vi "ParamSetAll.vi"(10 "error in (no error)":errorcluster caption="错误输入（无错误）") -> ()   [LabVIEW 2018]
panel:
  in  "确定":bool
  out "数值":i32
  out "原始数据":string[](array[string])=["general_param.vi", "PowerEnergyMeter_param.vi", "SpecMeter_param.vi", "Scope_param.vi", "Polarmeter_param.vi", "NearFieldCamera_param.vi", "FarFieldCamera_param.vi"]
  # "参数设置完成后，点击确定，参数下次运行会自动加载"
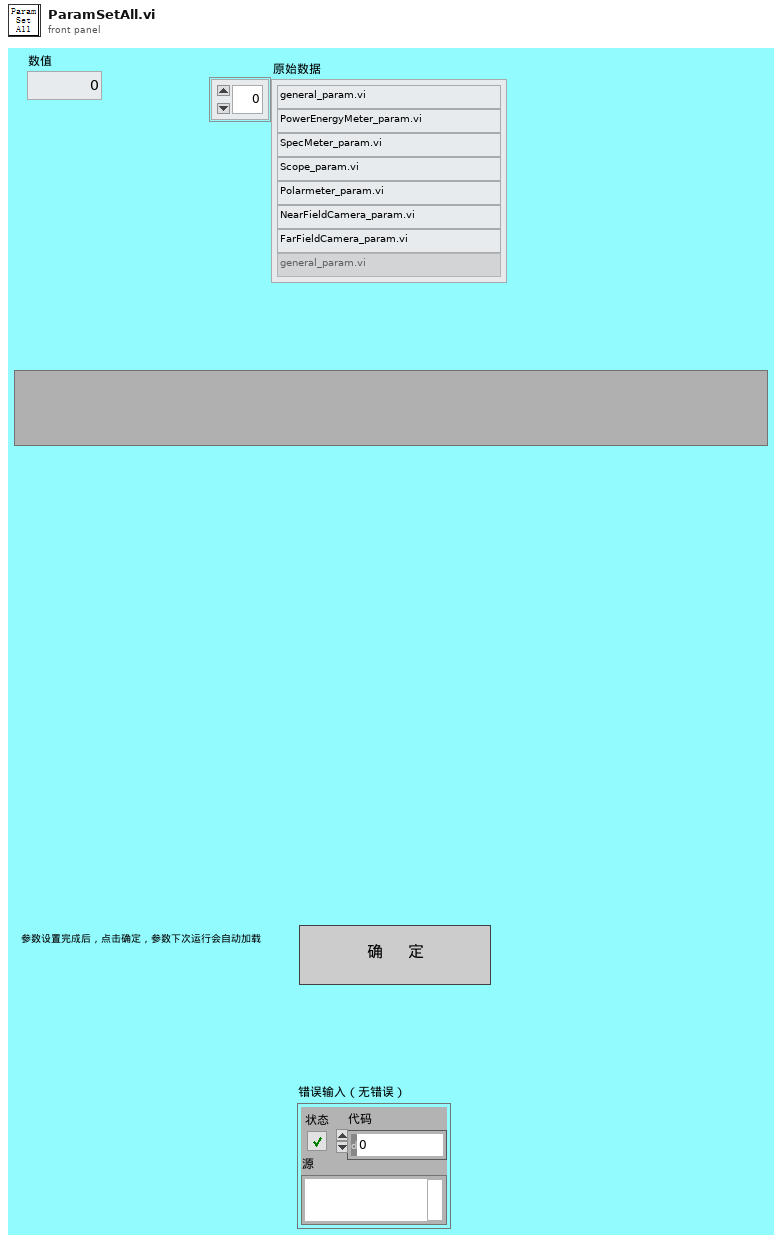
[diagram p1: front panel]
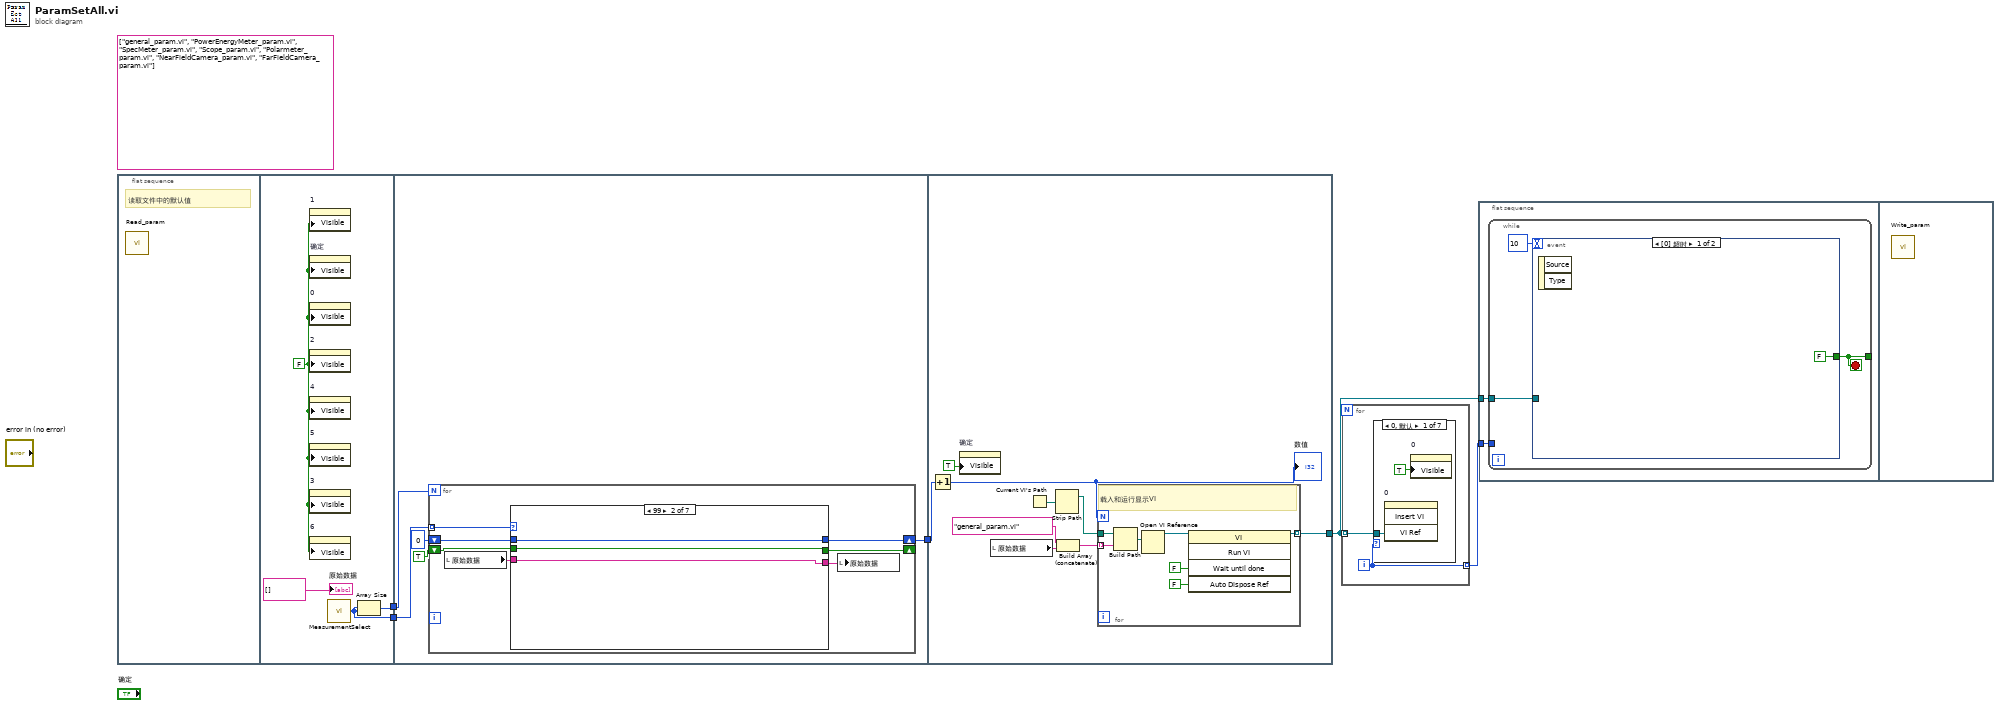
[diagram p0: block diagram]
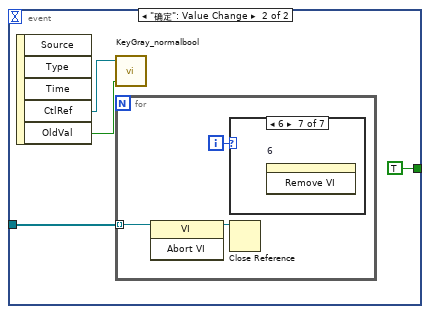
[diagram p2: hidden frame]
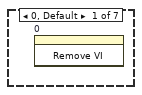
[diagram p3: hidden frame]
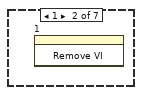
[diagram p4: hidden frame]
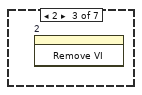
[diagram p5: hidden frame]
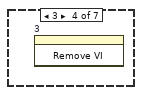
[diagram p6: hidden frame]
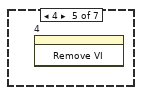
[diagram p7: hidden frame]
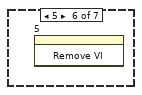
[diagram p8: hidden frame]
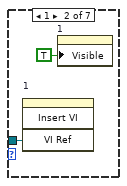
[diagram p9: hidden frame]
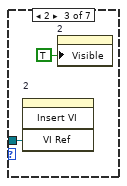
[diagram p10: hidden frame]
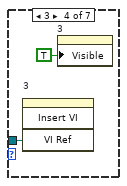
[diagram p11: hidden frame]
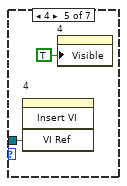
[diagram p12: hidden frame]
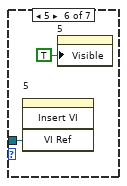
[diagram p13: hidden frame]
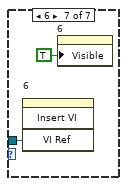
[diagram p14: hidden frame]
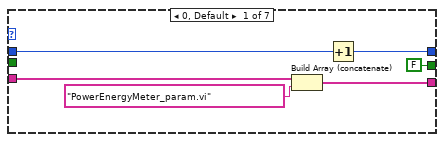
[diagram p15: hidden frame]
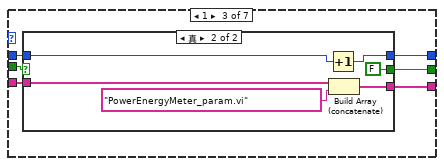
[diagram p16: hidden frame]
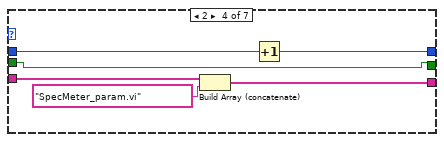
[diagram p18: hidden frame]
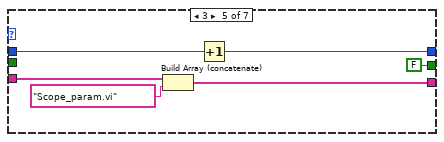
[diagram p19: hidden frame]
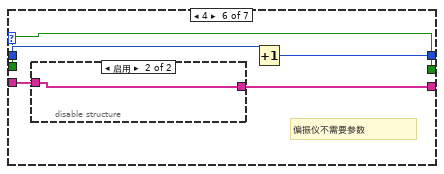
[diagram p20: hidden frame]
diagram:
  (unwired) string[] ["general_param.vi", "PowerEnergyMeter_param.vi", "SpecMeter_param.vi", "Scope_param.vi", "Polarmeter_param.vi", "NearFieldCamera_param.vi", "FarFieldCamera_param.vi"]
  n1 = flat-sequence {
    tunnel: [w8] -> w2
    tunnel: [w7] -> w1
    tunnel: [w12] -> w5
    tunnel: w2 -> [w11]
    tunnel: w1 -> [w10]
    tunnel: w5 -> [w81]
    tunnel: [w77] -> w3
    frame #0 {
      # "读取文件中的默认值"
      n2 = call "Read_param.vi"() -> ()  [unwired: 12 in]
    }
    frame #1 {
      w6 = FALSE
      n3 = property on="1" class="SubPnl"("Visible"=w6) -> ()  [unwired: 2 in, 2 out]
      n4 = property on="确定" class="Bool (严格)"("Visible"=w6) -> ()  [unwired: 2 in, 2 out]
      n5 = property on="0" class="SubPnl"("Visible"=w6) -> ()  [unwired: 2 in, 2 out]
      n6 = property on="2" class="SubPnl"("Visible"=w6) -> ()  [unwired: 2 in, 2 out]
      n7 = property on="4" class="SubPnl"("Visible"=w6) -> ()  [unwired: 2 in, 2 out]
      n8 = property on="5" class="SubPnl"("Visible"=w6) -> ()  [unwired: 2 in, 2 out]
      n9 = property on="3" class="SubPnl"("Visible"=w6) -> ()  [unwired: 2 in, 2 out]
      n10 = property on="6" class="SubPnl"("Visible"=w6) -> ()  [unwired: 2 in, 2 out]
      n11 = call "MeasurementSelect.vi"() -> ("任务序号"=w7:i32[])  [unwired: 1 in]
      n12 = Array Size(array=w7) -> (size(s)=w8:i32)
      "原始数据" <- string[] []
    }
    frame #2 {
      n13 = for {
        N: w11 -> [_]
        shift-right: [w20] -> _
        shift-left: TRUE -> [w21]
        shift-right: [w18] -> w12
        shift-left: 0 -> [w19]
        tunnel: w10 -> [w17] mode=indexing
        n14 = local read "原始数据"() -> (w15:string[])
        n15 = case shown="99" w17 {
          tunnel: w21 -> [_ w29 w36 w51 _ w60 w71]
          tunnel: [FALSE w29 w32 w51 FALSE w60 w71] -> w20
          tunnel: [w22 w30 w35 w46 w52 w58 w67] -> w16
          tunnel: w19 -> [w26 w28 w34 w50 w56 w62 w74]
          tunnel: [w25 w28 w33 w49 w55 w61 w72] -> w18
          tunnel: w15 -> [w24 w30 w31 w48 w54 w59 w70]
          frame 0, Default {
            n16 = Build Array (concatenate)(w24, "PowerEnergyMeter_param.vi" ("名称或相对路径")) -> (w22:string[])
            n17 = Increment(x=w26) -> (x+1=w25:i32)
          }
          frame 99 {
          }
          frame 1 {
            n18 = case shown="真" w36 {
              selector: w36 -> [w38 _]
              tunnel: [w37 w41] -> w35
              tunnel: [w39 w44] -> w33
              tunnel: w34 -> [w39 w45]
              tunnel: [w38 FALSE] -> w32
              tunnel: w31 -> [w37 w42]
              frame False {
              }
              frame True {
                n19 = Increment(x=w45) -> (x+1=w44:i32)
                n20 = Build Array (concatenate)(w42, "PowerEnergyMeter_param.vi" ("名称或相对路径")) -> (w41:string[])
              }
            }
          }
          frame 2 {
            n21 = Build Array (concatenate)(w48, "SpecMeter_param.vi" ("名称或相对路径")) -> (w46:string[])
            n22 = Increment(x=w50) -> (x+1=w49:i32)
          }
          frame 3 {
            n23 = Build Array (concatenate)(w54, "Scope_param.vi" ("名称或相对路径")) -> (w52:string[])
            n24 = Increment(x=w56) -> (x+1=w55:i32)
          }
          frame 4 {
            # "偏振仪不需要参数"
            n25 = disable-structure shown="启用" {
              disable-tunnel: w59 -> [w64 w66]
              disable-tunnel: [w63 w66] -> w58
              frame Disabled {
                n26 = Build Array (concatenate)(w64, "Polarmeter_param.vi" ("名称或相对路径")) -> (w63:string[])
              }
              frame Enabled {
              }
            }
            n27 = Increment(x=w62) -> (x+1=w61:i32)
          }
          frame 5 {
            n28 = Increment(x=w74) -> (x+1=w73:i32)
            n29 = Build Array (concatenate)(w70, "NearFieldCamera_param.vi" ("名称或相对路径"), "FarFieldCamera_param.vi" ("名称或相对路径")) -> (w67:string[])
            n30 = Increment(x=w73) -> (x+1=w72:i32)
          }
        }
        n31 = local write "原始数据"(w16) -> ()
      }
    }
    frame #3 {
      n32 = Increment(x=w81) -> (x+1=w76:i32)
      "数值" <- w76
      n33 = property on="确定" class="Bool (严格)"("Visible"=TRUE ("可见")) -> ()  [unwired: 2 in, 2 out]
      n34 = local read "原始数据"() -> (w80:string[])
      n35 = Current VI's Path() -> (path=w82:path)
      n36 = Strip Path(path=w82) -> (stripped path=w83:path)  [unwired: 1 out]
      n37 = Build Array (concatenate)("general_param.vi" ("名称或相对路径"), w80) -> (w79:string[])
      n38 = for {
        N: w76 -> [_]
        tunnel: [w84] -> w77 mode=indexing
        tunnel: w83 -> [w88]
        tunnel: w79 -> [w85] mode=indexing
        # "载入和运行显示VI"
        n39 = Build Path(base path=w88, name or relative path=w85) -> (appended path=w87:path)
        n40 = Open VI Reference(vi path=w87) -> (vi reference=w86:refnum<vi>)  [unwired: 5 in, 1 out]
        n41 = invoke on="Invoke Node" class="VI" method="Run VI"(reference=w86, "Wait until done"=FALSE ("Wait Until Done"), "Auto Dispose Ref"=FALSE ("Auto Dispose Reference")) -> (reference out=w84:refnum<vi>)  [unwired: 2 in, 4 out]
      }
    }
  }
  n42 = for {
    tunnel: w3 -> [w92] mode=indexing
    tunnel: [w91] -> w4 mode=indexing
    i -> [w91]
    n43 = case shown="0, 默认" w91 {
      tunnel: w92 -> [w94 w96 w98 w100 w102 w104 w106]
      frame 0, Default {
        n44 = invoke on="0" class="SubPnl" method="Insert VI"("VI Ref"=w94) -> ()  [unwired: 3 in, 4 out]
        n45 = property on="0" class="SubPnl"("Visible"=TRUE ("可见")) -> ()  [unwired: 2 in, 2 out]
      }
      frame 1 {
        n46 = invoke on="1" class="SubPnl" method="Insert VI"("VI Ref"=w96) -> ()  [unwired: 3 in, 4 out]
        n47 = property on="1" class="SubPnl"("Visible"=TRUE ("可见")) -> ()  [unwired: 2 in, 2 out]
      }
      frame 2 {
        n48 = invoke on="2" class="SubPnl" method="Insert VI"("VI Ref"=w98) -> ()  [unwired: 3 in, 4 out]
        n49 = property on="2" class="SubPnl"("Visible"=TRUE ("可见")) -> ()  [unwired: 2 in, 2 out]
      }
      frame 3 {
        n50 = invoke on="3" class="SubPnl" method="Insert VI"("VI Ref"=w100) -> ()  [unwired: 3 in, 4 out]
        n51 = property on="3" class="SubPnl"("Visible"=TRUE ("可见")) -> ()  [unwired: 2 in, 2 out]
      }
      frame 4 {
        n52 = invoke on="4" class="SubPnl" method="Insert VI"("VI Ref"=w102) -> ()  [unwired: 3 in, 4 out]
        n53 = property on="4" class="SubPnl"("Visible"=TRUE ("可见")) -> ()  [unwired: 2 in, 2 out]
      }
      frame 5 {
        n54 = invoke on="5" class="SubPnl" method="Insert VI"("VI Ref"=w104) -> ()  [unwired: 3 in, 4 out]
        n55 = property on="5" class="SubPnl"("Visible"=TRUE ("可见")) -> ()  [unwired: 2 in, 2 out]
      }
      frame 6 {
        n56 = invoke on="6" class="SubPnl" method="Insert VI"("VI Ref"=w106) -> ()  [unwired: 3 in, 4 out]
        n57 = property on="6" class="SubPnl"("Visible"=TRUE ("可见")) -> ()  [unwired: 2 in, 2 out]
      }
    }
  }
  n58 = flat-sequence {
    tunnel: w4 -> [w108]
    tunnel: w3 -> [w107]
    frame #0 {
      n59 = while {
        tunnel: w108 -> [_]
        tunnel: w107 -> [w110]
        tunnel: [w109] -> _
        stop <- w109 stop-if-true
        n60 = event shown="[0] 超时" {
          selector: _ -> [_ _]
          dyn-events: _ -> [_ _]
          timeout: 10 -> [_ _]
          tunnel: [FALSE TRUE] -> w109
          tunnel: w110 -> [_ w115]
          event Timeout {
            n61 = event-data() -> ()  [unwired: 1 in, 2 out]
          }
          event "确定": Value Change {
            n62 = event-data() -> ("CtlRef"=w114:refnum<vi>, "OldVal"=w113:bool)  [unwired: 1 in, 3 out]
            n63 = call "KeyGray_normalbool.vi"("OldVal"=w113, "引用"=w114) -> ()  [unwired: 2 in]
            n64 = for {
              tunnel: w115 -> [w119] mode=indexing
              i -> [w117]
              n65 = invoke class="VI" method="Abort VI"(reference=w119) -> (reference out=w118:refnum<vi>)  [unwired: 2 in, 2 out]
              n66 = case shown="6" w117 {
                frame 0, Default {
                  n67 = invoke on="0" class="SubPnl" method="Remove VI"() -> ()  [unwired: 3 in, 3 out]
                }
                frame 1 {
                  n68 = invoke on="1" class="SubPnl" method="Remove VI"() -> ()  [unwired: 3 in, 3 out]
                }
                frame 2 {
                  n69 = invoke on="2" class="SubPnl" method="Remove VI"() -> ()  [unwired: 3 in, 3 out]
                }
                frame 3 {
                  n70 = invoke on="3" class="SubPnl" method="Remove VI"() -> ()  [unwired: 3 in, 3 out]
                }
                frame 4 {
                  n71 = invoke on="4" class="SubPnl" method="Remove VI"() -> ()  [unwired: 3 in, 3 out]
                }
                frame 5 {
                  n72 = invoke on="5" class="SubPnl" method="Remove VI"() -> ()  [unwired: 3 in, 3 out]
                }
                frame 6 {
                  n73 = invoke on="6" class="SubPnl" method="Remove VI"() -> ()  [unwired: 3 in, 3 out]
                }
              }
              n74 = Close Reference(reference=w118) -> ()  [unwired: 1 in, 1 out]
            }
          }
        }
      }
    }
    frame #1 {
      n75 = call "Write_param.vi"() -> ()  [unwired: 12 in]
    }
  }
